vi "Time step.vi"(0 "Time (s)":dbl, 5 "Microwave on":bool=TRUE, 7 "Internal parameters in":T4, 9 "Fit parameters":T1, 11 "Physical constants":T3, 12 "System parameters":T2) -> (4 "Internal parameters out":T4, 15 "Fit parameters out":T1={"A"=0.572086, "S"=0.0835606, "M1"=140.286, "M2"=140.486})   [LabVIEW 2015]
uses:
  Internal Parameters.ctl
  Physical Constants.ctl
  System parameters.ctl
  Fit Parameters.ctl
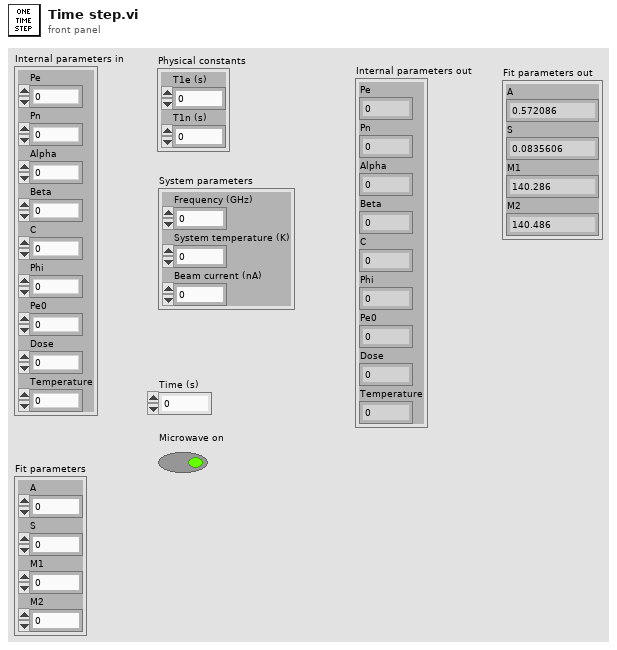
[diagram p1: front panel]
types:
  T1 = typedef "Fit Parameters.ctl" = cluster{"A":dbl, "S":dbl, "M1":dbl, "M2":dbl}
  T2 = typedef "System parameters.ctl" = cluster{"Frequency (GHz)":dbl, "System temperature (K)":dbl, "Beam current (nA)":dbl}
  T3 = typedef "Physical Constants.ctl" = cluster{"T1e (s)":dbl, "T1n (s)":dbl}
  T4 = typedef "Internal Parameters.ctl" = cluster{"Pe":dbl, "Pn":dbl, "Alpha":dbl, "Beta":dbl, "C":dbl, "Phi":dbl, "Pe0":dbl, "Dose":dbl, "Temperature":dbl}
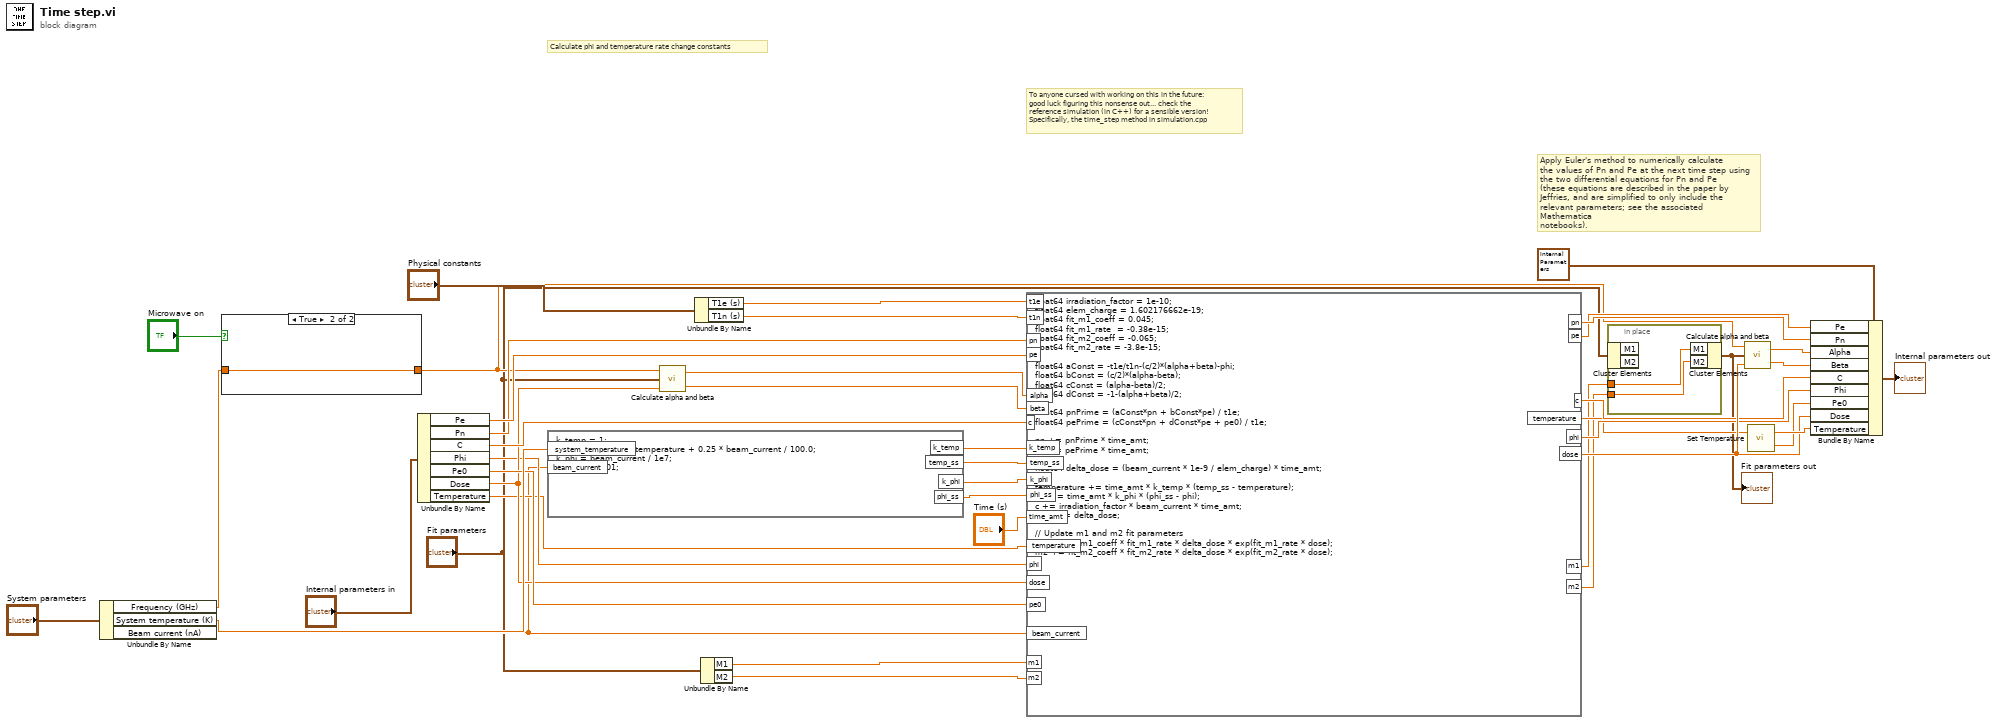
[diagram p0: block diagram]
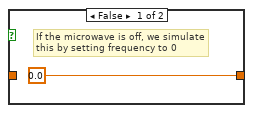
[diagram p2: hidden frame]
diagram:
  # "To anyone cursed with working on this in the future:\ngood luck figuring this nonsense out... check the\nreference simulation (in C++) for a sensible version!\nSpecifically, the time_step method in simulation.cpp"
  # "Apply Euler's method to numerically calculate\nthe values of Pn and Pe at the next time step using\nthe two differential equations for Pn and Pe\n(these equations are described in the paper by\nJeffries, and are simplified to only include the\nrelevant parameters; see the associated Mathematica\nnotebooks)."
  # "Calculate phi and temperature rate change constants"
  n1 = Unbundle By Name("System parameters") -> ("Frequency (GHz)"=w9:dbl, "System temperature (K)"=w32:dbl, "Beam current (nA)"=w22:dbl)
  n2 = case shown="True" "Microwave on" {
    tunnel: w9 -> [_ w44]
    tunnel: [0.0 ("Frequency") w44] -> w8
    frame False {
      # "If the microwave is off, we simulate\nthis by setting frequency to 0"
    }
    frame True {
    }
  }
  n3 = Unbundle By Name("Internal parameters in") -> ("Pe"=w29:dbl, "Pn"=w28:dbl, "C"=w27:dbl, "Phi"=w24:dbl, "Pe0"=w26:dbl, "Dose"=w25:dbl, "Temperature"=w23:dbl)
  n4 = formula code="k_temp = 1;\ntemp_ss = system_temperature + 0.25 * beam_current / 100.0;\nk_phi = beam_current / 1e7;\nphi_ss = 0.001;"("system_temperature"=w32, "beam_current"=w22) -> ("k_temp"=w42:dbl, "temp_ss"=w41:dbl, "k_phi"=w40:dbl, "phi_ss"=w39:dbl)
  n5 = call "Calculate alpha and beta.vi"("Dose"=w25, "Fit parameters"="Fit parameters", "Frequency (GHz)"=w8) -> ("Beta"=w37:dbl, "Alpha"=w38:dbl)
  n6 = Unbundle By Name("Physical constants") -> ("T1e (s)"=w31:dbl, "T1n (s)"=w30:dbl)
  n7 = Unbundle By Name("Fit parameters") -> ("M1"=w6:dbl, "M2"=w5:dbl)
  n8 = formula code="float64 irradiation_factor = 1e-10;\nfloat64 elem_charge = 1.602176662e-19;\nfloat64 fit_m1_coeff = 0.045;\nfloat64 fit_m1_rate  = -0.38e-15;\nfloat64 fit_m2_coeff = -0.065;\nfloat64 fit_m2_rate = -3.8e-15;\n\nfloat64 aConst = -t1e/t1n-(c/2)*(alpha+beta)-phi;\nfloat64 bConst = (c/2)*(alpha-beta);\nfloat64 cConst = (alpha-beta)/2;\nfloat64 dConst = -1-(alpha+beta)/2;\n\nfloat64 pnPrime = (aConst*pn + bConst*pe) / t1e;\nfloat64 pePrime = (cConst*pn + dConst*pe + pe0) / t1e;\n\npn += pnPrime * time_amt;\npe += pePrime * time_amt;\n\nfloat64 delta_dose = (beam_current * 1e-9 / elem_charge) * time_amt;\n\ntemperature += time_amt * k_temp * (temp_ss - temperature);\nphi += time_amt * k_phi * (phi_ss - phi);\nc += irradiation_factor * beam_current * time_amt;\ndose += delta_dose;\n\n// Update m1 and m2 fit parameters\nm1 += fit_m1_coeff * fit_m1_rate * delta_dose * exp(fit_m1_rate * dose);\nm2 += fit_m2_coeff * fit_m2_rate * delta_dose * exp(fit_m2_rate * dose);"("pn"=w28, "pe"=w29, "t1e"=w31, "alpha"=w38, "beta"=w37, "c"=w27, "t1n"=w30, "k_temp"=w42, "temp_ss"=w41, "k_phi"=w40, "phi_ss"=w39, "temperature"=w23, "time_amt"="Time (s)", "phi"=w24, "dose"=w25, "pe0"=w26, "beam_current"=w22, "m1"=w6, "m2"=w5) -> ("pn"=w12:dbl, "pe"=w11:dbl, "temperature"=w7:dbl, "phi"=w16:dbl, "dose"=w18:dbl, "c"=w15:dbl, "m1"=w3:dbl, "m2"=w2:dbl)
  n9 = in-place {
    in-place-border: w3 -> [w46]
    in-place-border: w2 -> [w45]
    n10 = in-place-cluster #1("Fit parameters") -> ()  [unwired: 2 out]
    n11 = in-place-cluster #1("M1"=w46, "M2"=w45) -> (w1:T1)
  }
  "Fit parameters out" <- w1
  n12 = call "Calculate alpha and beta.vi"("Dose"=w18, "Fit parameters"=w1, "Frequency (GHz)"=w8) -> ("Beta"=w13:dbl, "Alpha"=w14:dbl)
  n13 = call "Set Temperature.vi"("Temperature in"=w7) -> ("Pe0 out"=w17:dbl, "Temperature out"=w19:dbl)  [unwired: 1 in]
  n14 = Bundle By Name(cluster=T4 {"Pe"=0.0, "Pn"=0.0, "Alpha"=0.0, "Beta"=0.0, "C"=0.0, "Phi"=0.0, "Pe0"=0.0, "Dose"=0.0, "Temperature"=0.0} ("Simulation parameters out"), "Pe"=w11, "Pn"=w12, "Alpha"=w14, "Beta"=w13, "C"=w15, "Phi"=w16, "Pe0"=w17, "Dose"=w18, "Temperature"=w19) -> (→"Internal parameters out":T4)
